vi "Set Torque Setpoint.vi"(8 "error in (no error)":errorcluster, 10 "CCW torque (Nm)":dbl, 11 "NI_Robotics_KUKA youBot Arm Motor_Sim in":refnum<class "NI_Robotics_KUKA youBot Arm Motor_Sim.lvclass">) -> (0 "error out":errorcluster, 3 "NI_Robotics_KUKA youBot Arm Motor_Sim out":refnum<class "NI_Robotics_KUKA youBot Arm Motor_Sim.lvclass">)   [LabVIEW 2017, in "NI_Robotics_KUKA youBot Host.lvlib" / "NI_Robotics_KUKA youBot Arm Motor_Sim.lvclass"]
uses:
  <vilib>/robotics/KUKA youBot/Motor/Arm Motor Sim/NI_Robotics_KUKA youBot Arm Motor_Sim.lvclass
  <vilib>/robotics/KUKA youBot/Motor/Arm Motor Sim/NI_Robotics_KUKA youBot Arm Motor_Sim.lvclass/NI_Robotics_KUKA youBot Arm Motor_Sim.ctl
  <vilib>/robotics/Simulator/Robot Factory/Motor/ODESimulator_Motor.lvclass
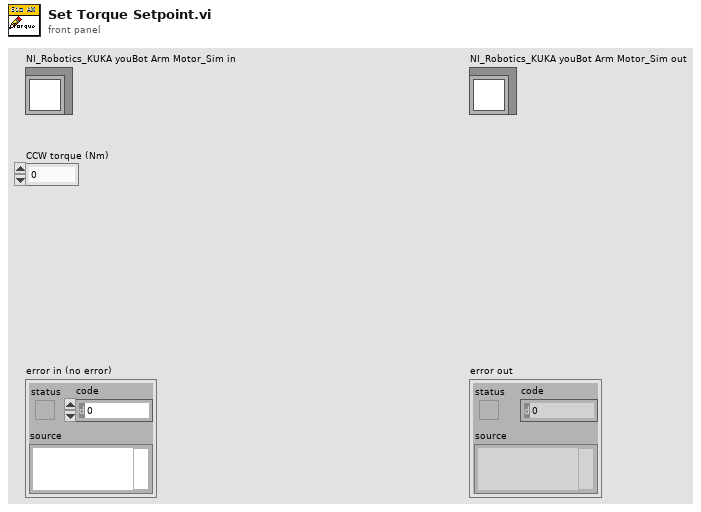
[diagram p1: front panel]
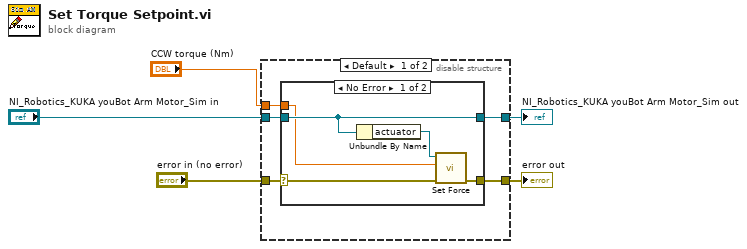
[diagram p0: block diagram]
diagram:
  n1 = disable-structure shown="Default" {
    disable-tunnel: "error in (no error)" -> [w10 w18]
    disable-tunnel: "CCW torque (Nm)" -> [w9 _]
    disable-tunnel: "NI_Robotics_KUKA youBot Arm Motor_Sim in" -> [w8 w19]
    disable-tunnel: [w7 w18] -> w1
    disable-tunnel: [w6 w19] -> w2
    frame condition #0 (active) {
      n2 = case shown="No Error" w10 {
        selector: w10 -> [w13 w16]
        tunnel: w9 -> [w11 _]
        tunnel: w8 -> [w15 w17]
        tunnel: [w12 w16] -> w7
        tunnel: [w15 w17] -> w6
        frame No Error {
          n3 = Unbundle By Name(w15) -> ("actuator"=w14:refnum<class "ODESimulator_Motor.lvclass">)
          n4 = call-dynamic "Set Force.vi"("error in (no error)"=w13, "force"=w11, "ODESimulator_Motor in"=w14) -> ("error out"=w12:errorcluster)  [unwired: 7 in, 1 out]
        }
        frame Error {
        }
      }
    }
    frame condition #1 {
    }
  }
  "error out" <- w1
  "NI_Robotics_KUKA youBot Arm Motor_Sim out" <- w2
